vi "Tracking.vi"() -> ()   [LabVIEW 2018]
doc: "The myRIO Project template acquires acceleration data from the onboard accelerometer and displays the changes of acceleration values in a waveform chart."
uses:
  <vilib>/myRIO/Instrument Drivers/Onboard IO/I2C/typedefs/I2C User Configuration.ctl
  <vilib>/myRIO/Instrument Drivers/Onboard IO/I2C/typedefs/I2C Transfer Rate.ctl
  <vilib>/myRIO/Instrument Drivers/Onboard IO/I2C/typedefs/I2C Reference.ctl
  <vilib>/myRIO/Common/Instrument Driver Framework/Utilities/typedefs/myRIO Generic Hardware Reference.ctl
  <vilib>/myRIO/Common/Instrument Driver Framework/Utilities/typedefs/Hardware Version Enum.ctl
  <vilib>/myRIO/Common/Instrument Driver Framework/Utilities/typedefs/myRIO v1.0 Reference.ctl
  <vilib>/myRIO/Common/Instrument Driver Framework/Utilities/typedefs/Generic FPGA Reference.ctl
  <vilib>/myRIO/Common/Instrument Driver Framework/myRIO v1.0/I2C/typedefs/I2C Channels Enum.ctl
  <vilib>/myRIO/Instrument Drivers/Onboard IO/I2C/typedefs/I2C Configuration.ctl
  <vilib>/userdefined/High Color/nirio_resource_hc.ctl
  <vilib>/myRIO/Common/Instrument Driver Framework/Utilities/vis/Is FPGA Ref Available.vi
  <vilib>/myRIO/Common/Instrument Driver Framework/myRIO v1.0/I2C/vis/myRIO v1.1 Open I2C.vi
  <vilib>/myRIO/Instrument Drivers/Onboard IO/I2C/vis/Configure.vi
  <vilib>/myRIO/Instrument Drivers/Onboard IO/I2C/vis/Read.vi
  <vilib>/myRIO/Common/Instrument Driver Framework/myRIO v1.0/PWM/vis/myRIO v1.1 Open PWM.vi
  <vilib>/myRIO/Common/Instrument Driver Framework/Utilities/vis/Validate Channels.vi
  <vilib>/myRIO/Common/Instrument Driver Framework/myRIO v1.0/I2C/vis/myRIO v1.0 Reserve I2C.vi
  <vilib>/myRIO/Common/Instrument Driver Framework/myRIO v1.0/UART/vis/myRIO v1.0 Close UART.vi
  <vilib>/myRIO/Common/Instrument Driver Framework/myRIO v1.0/PWM/vis/myRIO v1.0 Reserve PWM.vi
  <vilib>/myRIO/Common/Instrument Driver Framework/myRIO v1.0/I2C/vis/myRIO v1.0 Build MUX Configuration I2C.vi
  <vilib>/myRIO/Common/Instrument Driver Framework/myRIO v1.0/Resource Manager/vis/myRIO v1.0 Reserve Channel List.vi
  <vilib>/myRIO/Common/Instrument Driver Framework/myRIO v1.0/PWM/vis/myRIO v1.0 Build MUX Configuration PWM.vi
  <vilib>/myRIO/Common/Instrument Driver Framework/myRIO v1.0/Resource Manager/vis/myRIO v1.0 Create Configuration List.vi
  <vilib>/myRIO/Common/Instrument Driver Framework/myRIO v1.0/Resource Manager/vis/myRIO v1.0 Reserve Channel.vi
  <vilib>/myRIO/Common/Instrument Driver Framework/myRIO v1.0/Resource Manager/vis/myRIO v1.0 Unreserve Channel.vi
  <vilib>/myRIO/Common/Instrument Driver Framework/myRIO v1.0/Resource Manager/vis/myRIO v1.0 Build Mutex Name.vi
  <vilib>/Utility/VariantDataType/GetNumericInfo.vi
  <vilib>/Utility/error.llb/Error Cluster From Error Code.vi
  <vilib>/myRIO/Common/Instrument Driver Framework/myRIO v1.0/myRIO v1.1 Open.vi
  <vilib>/myRIO/Common/Instrument Driver Framework/Utilities/vis/IO Manager.vi
  <vilib>/myRIO/Common/Instrument Driver Framework/Utilities/vis/Configuration Manager.vi
  <vilib>/myRIO/Common/Instrument Driver Framework/myRIO v1.0/Resource Manager/vis/myRIO v1.0 Configure IO.vi
  <vilib>/myRIO/Common/Instrument Driver Framework/myRIO v1.0/myRIO v1.0 Close.vi
  <vilib>/myRIO/Common/Instrument Driver Framework/myRIO v1.0/I2C/vis/myRIO v1.0 Configure I2C.vi
  <vilib>/myRIO/Common/Instrument Driver Framework/myRIO v1.0/I2C/vis/myRIO v1.0 Read I2C.vi
  <vilib>/myRIO/Common/Instrument Driver Framework/myRIO v1.0/PWM/vis/myRIO v1.0 Write PWM.vi
  <vilib>/myRIO/Common/Instrument Driver Framework/Utilities/vis/FPGA Ref Manager.vi
  <vilib>/myRIO/Common/Instrument Driver Framework/myRIO v1.0/myRIO v1.0 Reset FPGA.vi
  <vilib>/myRIO/Common/Instrument Driver Framework/myRIO v1.0/IRQ/vis/myRIO v1.0 IRQ Info FGV.vi
  <vilib>/myRIO/Common/Instrument Driver Framework/myRIO v1.0/IRQ/vis/myRIO v1.0 Timer IRQ Info FGV.vi
  <vilib>/myRIO/Common/Instrument Driver Framework/myRIO v1.0/IRQ/vis/myRIO v1.0 ISR Agent.vi
  <vilib>/myRIO/Express VI/Onboard IO/I2C/I2C Express VI.xnode
  <vilib>/myRIO/Instrument Drivers/Onboard IO/I2C/vis/myRIO I2C Open.xnode
  <vilib>/myRIO/Instrument Drivers/Onboard IO/I2C/I2C.lvlib
  <vilib>/myRIO/Instrument Drivers/Onboard IO/PWM/PWM.lvlib
  <vilib>/myRIO/Instrument Drivers/Utilities/Utilities.lvlib
panel:
  in  "KDy":dbl
  in  "KDx":dbl
  in  "position y 2":dbl(slide)=90.0 scale=0.0..100.0
  in  "position x 2":dbl(slide)=90.0 scale=0.0..180.0
  in  "stop":bool
  in  "control":bool
  out "x":i32
  out "y":i32
  out "position x":dbl(slide) scale=0.0..180.0
  out "position y":dbl(slide) scale=0.0..120.0
  in  "PWM y":tag="B/PWM0"
  in  "PWM x":tag="B/PWM0"
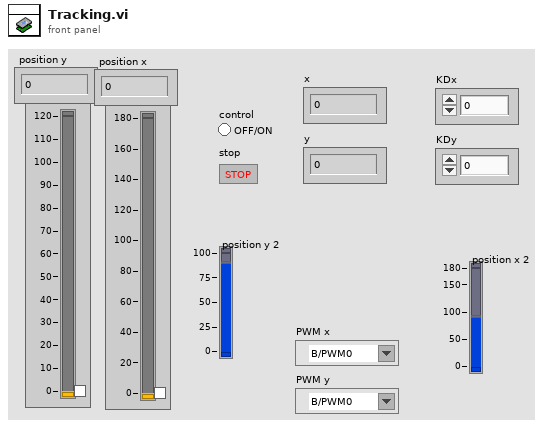
[diagram p1: front panel]
types:
  T1 = typedef "PWM.lvlib/PWM Reference.ctl" = cluster{"myRIO Reference":T2, "PWM Channels Enum":T6, "PWM Configuration":T7}
  T2 = typedef "myRIO Generic Hardware Reference.ctl" = cluster{"myRIO Model":T3, "myRIO Hardware Reference":T4}
  T3 = typedef "Hardware Version Enum.ctl" = enum16{"Unknown", "myRIO-1900", "myRIO-1950", "roboRIO", "NI ELVIS RIO CM", "ELVIS III"}
  T4 = typedef "myRIO v1.0 Reference.ctl" = cluster{"Generic FPGA Reference":T5, "Allow multiple opens":bool}
  T5 = typedef "Generic FPGA Reference.ctl" = refnum<k20>
  T6 = typedef "PWM Channels Enum.ctl" = enum16{"Not Connected", "C/PWM0", "C/PWM1", "A/PWM0", "A/PWM1", "A/PWM2", "A/PWM3", "A/PWM4", "A/PWM5", "A/PWM6", "A/PWM7", "A/PWM8", "A/PWM9", "A/PWM10", "A/PWM11", "A/PWM12", "A/PWM13", "A/PWM14", "A/PWM15", "A/PWM16", "A/PWM17", "A/PWM18", "A/PWM19", "B/PWM0", "B/PWM1", "B/PWM2", "B/PWM3", "B/PWM4", "B/PWM5", "B/PWM6", "B/PWM7", "B/PWM8", "B/PWM9", "B/PWM10", "B/PWM11", "B/PWM12", "B/PWM13", "B/PWM14", "B/PWM15", "B/PWM16", "B/PWM17", "B/PWM18", "B/PWM19", "PWM/PWM0", "PWM/PWM1", "PWM/PWM2", "PWM/PWM3", "PWM/PWM4", "PWM/PWM5", "PWM/PWM6", "PWM/PWM7", "PWM/PWM8", "PWM/PWM9"}
  T7 = typedef "PWM.lvlib/PWM Configuration.ctl" = cluster{"Frequency":dbl, "Duty Cycle":dbl}
  T8 = typedef "I2C.lvlib/I2C Reference.ctl" = cluster{"myRIO Reference":T2, "I2C Channels Enum":T9, "I2C Configuration":T10}
  T9 = typedef "I2C Channels Enum.ctl" = enum16{"Not Connected", "A/I2C", "B/I2C", "I2C/I2C"}
  T10 = typedef "I2C.lvlib/I2C Configuration.ctl" = cluster{"I2C Transfer Rate":T11}
  T11 = typedef "I2C.lvlib/I2C Transfer Rate.ctl" = enum16{"Standard mode (100 kbps)", "Fast mode (400 kbps)"}
  T12 = typedef "I2C.lvlib/I2C User Configuration.ctl" = cluster{"I2C Transfer Rate":T11}
  T13 = typedef "nirio_resource_hc.ctl" = tag
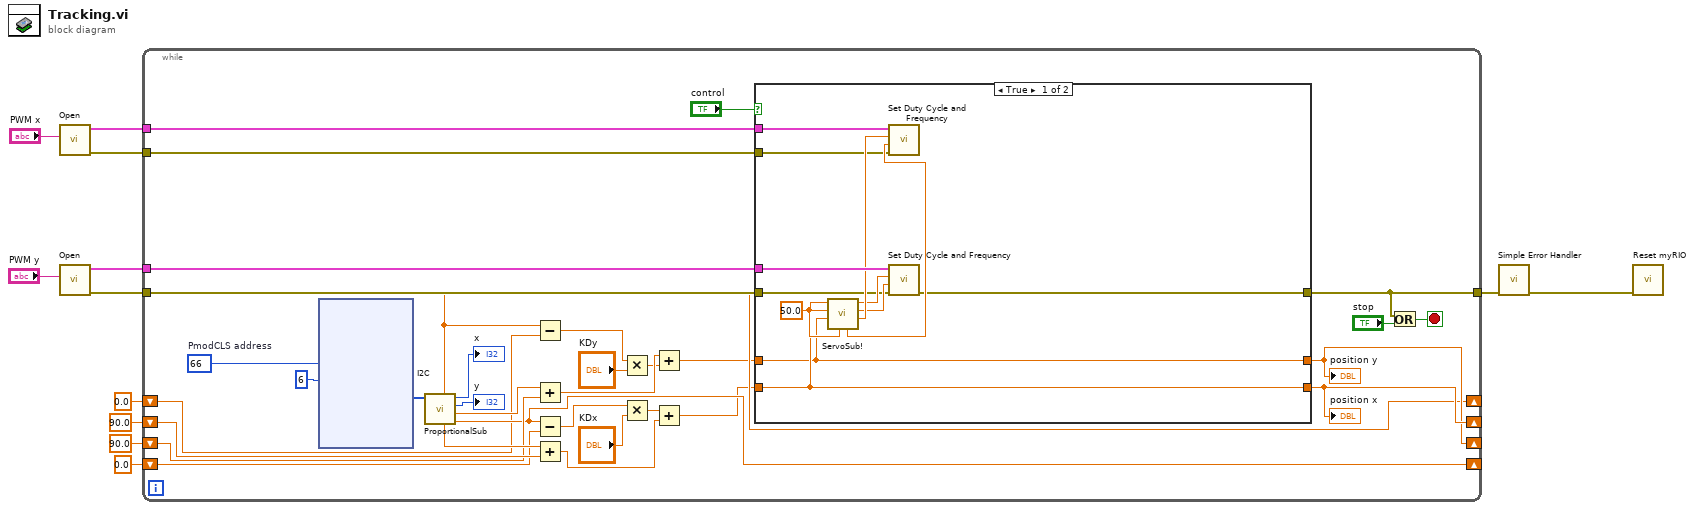
[diagram p0: block diagram]
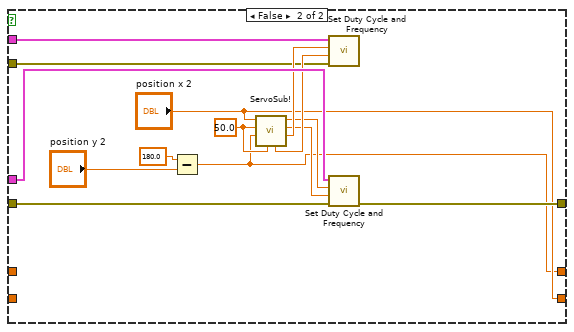
[diagram p2: hidden frame]
diagram:
  n1 = call <vilib>:"Open.vi"("Channel Name"="PWM x") -> ("error out"=w7:errorcluster, "PWM Ref Out"=w10:T1)  [unwired: 9 in]
  n2 = call <vilib>:"Open.vi"("Channel Name"="PWM y") -> ("error out"=w8:errorcluster, "PWM Ref Out"=w9:T1)  [unwired: 9 in]
  n3 = while {
    tunnel: w10 -> [w44]
    tunnel: w9 -> [w43]
    tunnel: w8 -> [w42]
    tunnel: w7 -> [w41]
    tunnel: [w25] -> w5
    shift-right: [w30] -> _
    shift-left: 90.0 -> [w35]
    shift-right: [w29] -> _
    shift-left: 90.0 -> [w34]
    shift-right: [w24] -> _
    shift-left: 0.0 -> [w23]
    shift-right: [w21] -> _
    shift-left: 0.0 -> [w22]
    stop <- w40 stop-if-true
    w38 = u8 66  # PmodCLS address
    n4 = xnode "I2C"("Slave Address (7-bit)"=w38, "Byte Count"=u32 6) -> ("Bytes Read"=w39:u8[])  [unwired: 1 in, 1 out]
    n5 = call "ProportionalSub.vi"("Bytes Read"=w39) -> ("XError"=w24:dbl, 1:"y"=w36:dbl, 2:"y"=→"y":i32, 3:"x"=→"x":i32, 4:"x"=w37:dbl, "YError"=w21:dbl)  [unwired: 5 in]
    n6 = Subtract(x=w21, y=w22) -> (x-y=w18:dbl)
    n7 = Add(x=w36, y=w34) -> (x+y=w31:dbl)
    n8 = Subtract(x=w24, y=w23) -> (x-y=w20:dbl)
    n9 = Add(x=w37, y=w35) -> (x+y=w32:dbl)
    n10 = Multiply(x=w18, y="KDy") -> (x*y=w15:dbl)
    n11 = Multiply(x=w20, y="KDx") -> (x*y=w13:dbl)
    n12 = Add(x=w31, y=w15) -> (x+y=w16:dbl)
    n13 = Add(x=w13, y=w32) -> (x+y=w14:dbl)
    n14 = case shown="True" "control" {
      tunnel: w44 -> [w57 w71]
      tunnel: w43 -> [w56 w70]
      tunnel: w42 -> [w50 w64]
      tunnel: w41 -> [w49 w63]
      tunnel: [w48 w62] -> w25
      tunnel: w14 -> [w47 _]
      tunnel: w16 -> [w46 _]
      tunnel: [w47 "position x 2"] -> w30
      tunnel: [w46 w59] -> w29
      frame True {
        w55 = 50.0 ("freq [Hz]")
        n15 = call "ServoSub!.vi"("freq [Hz] 2"=w55, "position [%FS] 2"=w46, "freq [Hz]"=w55, "position [%FS]"=w47) -> ("Numeric"=w53:dbl, "freq [Hz] 4"=w52:dbl, "Numeric 2"=w51:dbl, "freq [Hz] 3"=w54:dbl)  [unwired: 4 in]
        n16 = call <vilib>:"Set Duty Cycle and Frequency.vi"("error in (no error)"=w49, "Frequency [Hz]"=w54, "Duty Cycle"=w53, "PWM Ref In"=w57) -> ()  [unwired: 5 in, 2 out]
        n17 = call <vilib>:"Set Duty Cycle and Frequency.vi"("error in (no error)"=w50, "Frequency [Hz]"=w52, "Duty Cycle"=w51, "PWM Ref In"=w56) -> ("error out"=w48:errorcluster)  [unwired: 5 in, 1 out]
      }
      frame False {
        w69 = 50.0 ("freq [Hz]")
        n18 = Subtract(x=180.0, y="position y 2") -> (x-y=w59:dbl)
        n19 = call "ServoSub!.vi"("freq [Hz] 2"=w69, "position [%FS] 2"=w59, "freq [Hz]"=w69, "position [%FS]"="position x 2") -> ("Numeric"=w67:dbl, "freq [Hz] 4"=w66:dbl, "Numeric 2"=w65:dbl, "freq [Hz] 3"=w68:dbl)  [unwired: 4 in]
        n20 = call <vilib>:"Set Duty Cycle and Frequency.vi"("error in (no error)"=w63, "Frequency [Hz]"=w68, "Duty Cycle"=w67, "PWM Ref In"=w71) -> ()  [unwired: 5 in, 2 out]
        n21 = call <vilib>:"Set Duty Cycle and Frequency.vi"("error in (no error)"=w64, "Frequency [Hz]"=w66, "Duty Cycle"=w65, "PWM Ref In"=w70) -> ("error out"=w62:errorcluster)  [unwired: 5 in, 1 out]
      }
    }
    "position x" <- w30
    "position y" <- w29
    n22 = Or(x=w25, y="stop") -> (x .or. y?=w40:bool)
  }
  n23 = call <vilib>:"Simple Error Handler.vi"("error in (no error)"=w5) -> ("error out"=w6:errorcluster)  [unwired: 4 in, 4 out]
  n24 = call <vilib>:"Reset myRIO.vi"("error in (no error)"=w6) -> ()  [unwired: 10 in, 1 out]
